vi "GV ZstageAsTrigger.vi"() -> ()   [LabVIEW 2017]
panel:
  out "ZstageAsTrig":bool
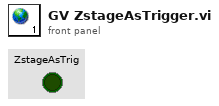
[diagram p1: front panel]
diagram:
